vi "task2_counter.vi"() -> ()   [LabVIEW 2020]
panel:
  in  "stop":bool
  in  "Reset Button":bool
  out "counter":dbl
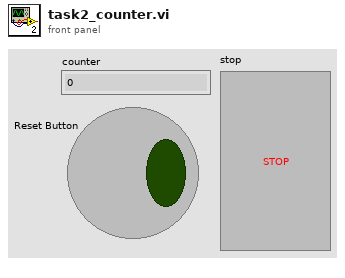
[diagram p1: front panel]
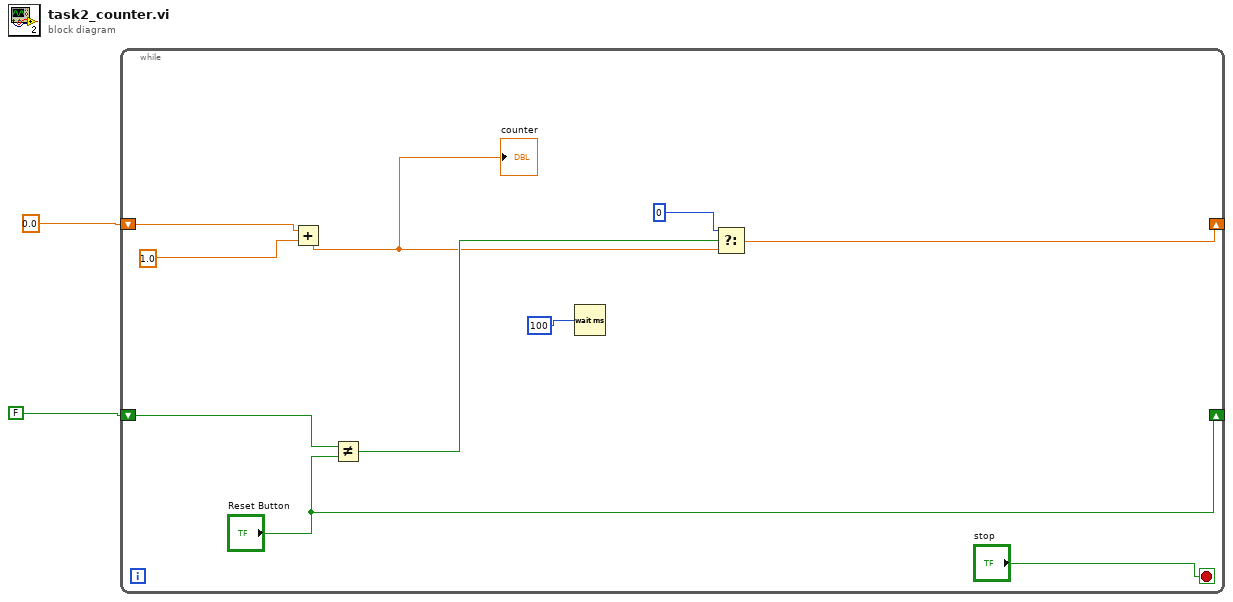
[diagram p0: block diagram]
diagram:
  n1 = while {
    shift-right: ["Reset Button"] -> _
    shift-left: FALSE -> [w12]
    shift-right: [w5] -> _
    shift-left: 0.0 -> [w10]
    stop <- "stop" stop-if-true
    n2 = Add(x=w10, y=1.0) -> (x+y=w7:dbl)
    "counter" <- w7
    n3 = Not Equal?(x=w12, y="Reset Button") -> (x != y?=w8:bool)
    n4 = Wait (ms)(milliseconds to wait=100) -> ()  [unwired: 1 out]
    n5 = Select(t=0, s=w8, f=w7) -> (s? t:f=w5:dbl)
  }
